vi "数组.vi"() -> ()   [LabVIEW 2018]
panel:
  out "数组 2":dbl[][](array[numeric])
  out "数组":dbl[](array[numeric])
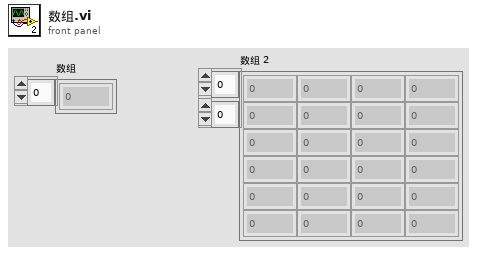
[diagram p1: front panel]
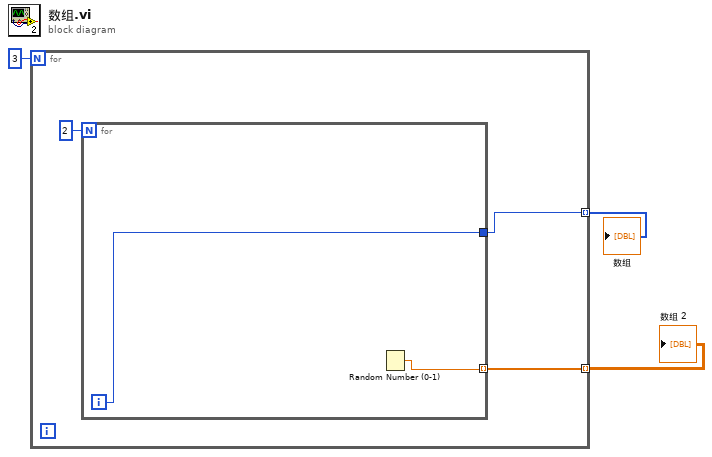
[diagram p0: block diagram]
diagram:
  n1 = for {
    N: 3 -> [_]
    tunnel: [w6] -> w3 mode=indexing
    tunnel: [w4] -> w1 mode=indexing
    n2 = for {
      N: 2 -> [_]
      tunnel: [w8] -> w4
      tunnel: [w7] -> w6 mode=indexing
      i -> [w8]
      n3 = Random Number (0-1)() -> (number: 0 to 1=w7:dbl)
    }
  }
  "数组 2" <- w3
  "数组" <- w1
